vi "Write Tags 2.vi"(8 "error in (no error)":errorcluster, 11 "State in":T1={"State"=enum."Measuring", "Start Time"=timestamp(0 s since 1904-01-01), "Current Time"=timestamp(0 s since 1904-01-01), "First Iteration"=FALSE, "Data"={"D-O State"=enum."Off"}, "Process Name"="", "Output Error"=FALSE, "Log Started"=FALSE, "Cycle Period"=0.0, "Configuration"={"Valve Settings"={"D-O Settings"={"DAQmx Task Name"="", "Output Channel"=0, "Output Channel Names"=[]}, "VICI Electronic Actuator"={"VISA resource name"="", "Mode"=enum."Two Positions With Stops", "Simulated"=FALSE}}, "Valve Type"=enum."Digital Output Valve", "Time On (Sec)"=0.0, "Time Off (Sec)"=0.0, "Run?"=FALSE}} {"Configuration"."Valve Settings"."D-O Settings"."Output Channel" items=["Choose a Channel"]}) -> (0 "error out":errorcluster)   [LabVIEW 2018, in "D-O Module.lvlib" / "D-O Module Engine.lvlib"]
uses:
  D-O Module Engine.lvlib
  State Cluster.ctl
  State Enum.ctl
  Valve Clusters.ctl
  D-O Module Settings Cluster.ctl
  D-O Device Settings Cluster.ctl
  VICI Electronic Actuator/VICI Electronic Actuator Settings.ctl
  Tag VIs/Tag FGV Operation Enum.ctl
  Shared Variables/Dynamic Shared Variables.lvlib
  D-O Module.lvlib
  DIO Valve/VICI Electronic Actuator.lvlib
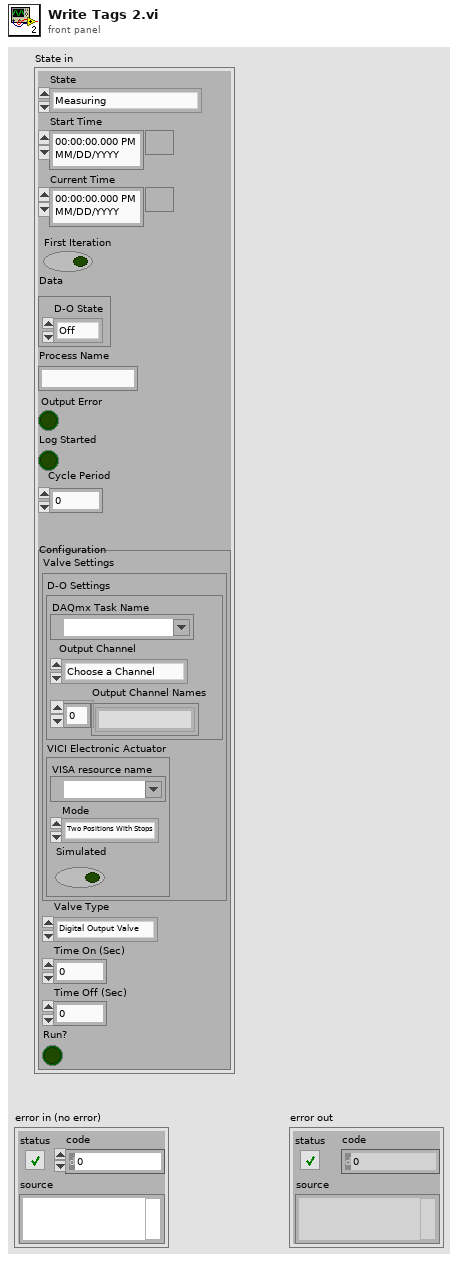
[diagram p1: front panel]
types:
  T1 = typedef "D-O Module.lvlib/D-O Module Engine.lvlib/State Cluster.ctl" = cluster{"State":T2, "Start Time":timestamp, "Current Time":timestamp, "First Iteration":bool, "Data":cluster{"D-O State":enum16{"Off", "On", "Not Initialized"}}, "Process Name":string, "Output Error":bool, "Log Started":bool, "Cycle Period":dbl, "Configuration":T3}
  T2 = typedef "D-O Module.lvlib/D-O Module Engine.lvlib/State Enum.ctl" = enum16{"Measuring", "Idle", "Paused"}
  T3 = typedef "D-O Module.lvlib/Valve Clusters.ctl" = cluster{"Valve Settings":T4, "Valve Type":enum16{"Default", "Digital Output Valve", "VICI Electronic Actuator"}, "Time On (Sec)":dbl, "Time Off (Sec)":dbl, "Run?":bool}
  T4 = typedef "D-O Module.lvlib/D-O Module Settings Cluster.ctl" = cluster{"D-O Settings":T5, "VICI Electronic Actuator":T6}
  T5 = typedef "D-O Module.lvlib/D-O Device Settings Cluster.ctl" = cluster{"DAQmx Task Name":refnum<k21>, "Output Channel":u16, "Output Channel Names":string[]}
  T6 = typedef "VICI Electronic Actuator.lvlib/VICI Electronic Actuator Settings.ctl" = cluster{"VISA resource name":refnum<visa-resource-name>, "Mode":enum16{"Two Positions With Stops", "Two Positions Without Stops", "Mutiposition"}, "Simulated":bool}
  T7 = typedef "Tag FGV Operation Enum.ctl" = enum16{"Init", "Set Notification Queue", "Create Tag", "Commit", "Write Tag (Numeric)", "Write Tag (Boolean)", "Read All Tags", "Read One Tag", "Delete Tag Category", "Set Alarm Parameters (Numeric)", "Set Alarm Parameters (Boolean)", "Enable All Alarms", "Disable All Alarms", "Delete All Tags", "Read Alarms", "Ack Alarm", "Read Alarm Parameters (Numeric)", "Read Alarm Parameters (Boolean)"}
  T8 = enum16{"Default", "Digital Output Valve", "VICI Electronic Actuator"}
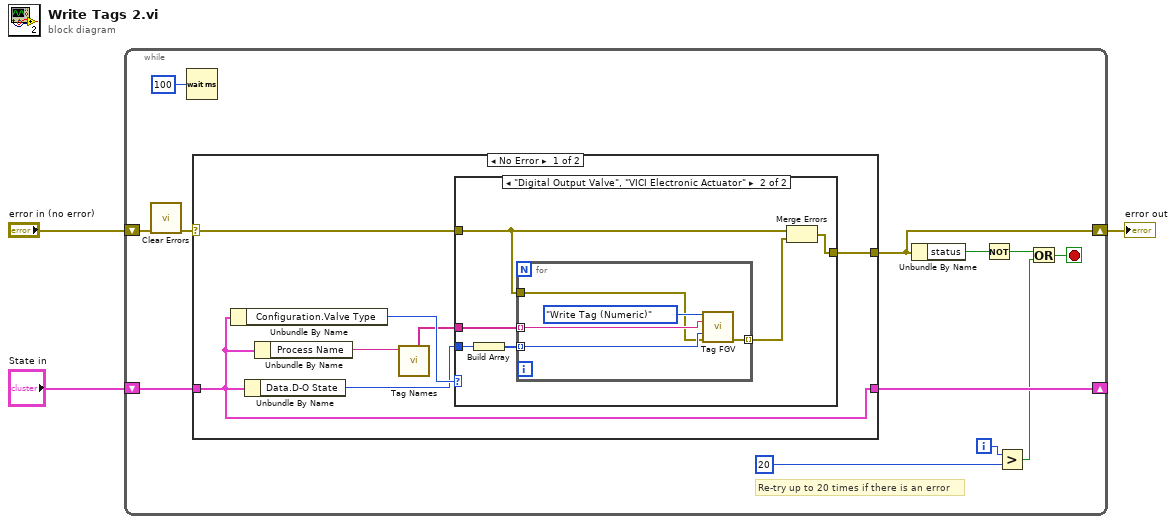
[diagram p0: block diagram]
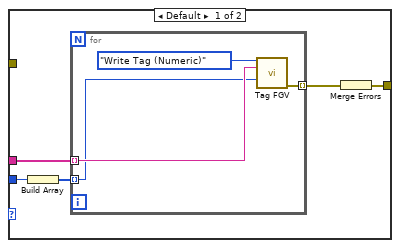
[diagram p2: hidden frame]
diagram:
  n1 = while {
    shift-right: [w9] -> w3
    shift-left: "error in (no error)" -> [w7]
    shift-right: [w14] -> _
    shift-left: "State in" -> [w15]
    i -> [w5]
    stop <- w13 stop-if-true
    # "Re-try up to 20 times if there is an error"
    n2 = call <vilib>:"Clear Errors.vi"("error in (no error)"=w7) -> ("error out"=w6:errorcluster)  [unwired: 5 in, 1 out]
    n3 = Wait (ms)(milliseconds to wait=u32 100) -> ()  [unwired: 1 out]
    n4 = case shown="No Error" w6 {
      selector: w6 -> [w19 w44]
      tunnel: [w20 w44] -> w9
      tunnel: w15 -> [w16 w43]
      tunnel: [w16 w43] -> w14
      frame No Error {
        n5 = Unbundle By Name(w16) -> ("Configuration.Valve Type"=w22:T8)
        n6 = Unbundle By Name(w16) -> ("Data.D-O State"=w21:enum16{"Off", "On", "Not Initialized"})
        n7 = Unbundle By Name(w16) -> ("Process Name"=w18:string)
        n8 = call "Tag Names.vi"("Process Name"=w18) -> ("All  Numeric Tags"=w17:string[])  [unwired: 8 in, 2 out]
        n9 = case shown="\"Digital Output Valve\", \"VICI Electronic Actuator\"" w22 {
          tunnel: w17 -> [w27 w35]
          tunnel: w21 -> [w23 w36]
          tunnel: [w24 w32] -> w20
          tunnel: w19 -> [_ w33]
          frame Default {
            n10 = Build Array(w23) -> (w26:enum16{"Off", "On", "Not Initialized"}[])
            n11 = for {
              tunnel: w27 -> [w30] mode=indexing
              tunnel: w26 -> [w29] mode=indexing
              tunnel: [w28] -> w25 mode=indexing
              n12 = call "Tag FGV.vi"("Operation"=Tag_FGV_Operation_Enum."Write Tag (Numeric)", "Tag Name"=w30, "Data"=w29) -> ("error out"=w28:errorcluster)  [unwired: 5 in, 7 out]
            }
            n13 = Merge Errors(w25) -> (w24:errorcluster)
          }
          frame "Digital Output Valve", "VICI Electronic Actuator" {
            n14 = Build Array(w36) -> (w37:enum16{"Off", "On", "Not Initialized"}[])
            n15 = for {
              tunnel: w37 -> [w41] mode=indexing
              tunnel: [w38] -> w34 mode=indexing
              tunnel: w35 -> [w40] mode=indexing
              tunnel: w33 -> [w39]
              n16 = call "Tag FGV.vi"("Operation"=Tag_FGV_Operation_Enum."Write Tag (Numeric)", "Tag Name"=w40, "Data"=w41, "error in (no error)"=w39) -> ("error out"=w38:errorcluster)  [unwired: 4 in, 7 out]
            }
            n17 = Merge Errors(w33, w34) -> (w32:errorcluster)
          }
        }
      }
      frame Error {
      }
    }
    n18 = Unbundle By Name(w9) -> ("status"=w8:bool)
    n19 = Not(x=w8) -> (.not. x?=w12:bool)
    n20 = Greater?(x=w5, y=20) -> (0:w10:bool)
    n21 = Or(x=w12, y=w10) -> (x .or. y?=w13:bool)
  }
  "error out" <- w3
